vi "Get Plot to Fit.vi"(8 "error in (no error)":errorcluster, 9 "Plot Index":i32, 11 "XYGraph in":T2) -> (0 "error out":errorcluster, 1 "Plot Name":string, 2 "Y Array out":dbl[](array[numeric]), 3 "X Array out":dbl[](array[numeric]), 4 "Plot Color":u32, 5 "(Clipped) Plot Range":T1, 7 "Plot clipped?":bool)   [LabVIEW 2019]
uses:
  Graphs/XY Graph/XY Graph Refnum.ctl
  Graphs/Plot Range.ctl
  Histograms/Histogram Window.lvlib
  Graphs/XY Graph/XY Graph Add-Ons.lvlib
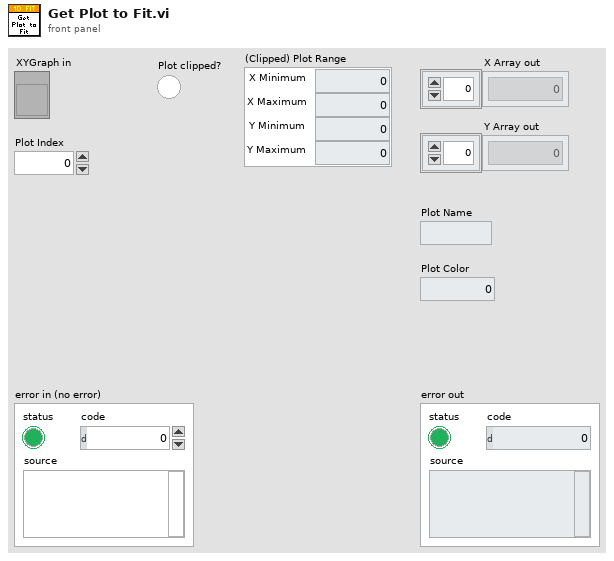
[diagram p1: front panel]
types:
  T1 = typedef "Plot Range.ctl" = cluster{"X Minimum":dbl, "X Maximum":dbl, "Y Minimum":dbl, "Y Maximum":dbl}
  T2 = typedef "XY Graph Add-Ons.lvlib/XY Graph Refnum.ctl" = refnum<vi>
  T3 = typedef "Histogram Bin Position.ctl" = enum16{"Left", "Center", "Right"}
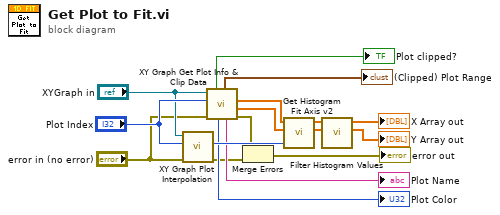
[diagram p0: block diagram]
diagram:
  n1 = call "XY Graph Plot Interpolation.vi"("error in (no error)"="error in (no error)", "Active Plot"="Plot Index", "XYGraph in"="XYGraph in") -> ("error out"=w3:errorcluster, "Bin Location"=w17:T3)  [unwired: 6 in, 1 out]
  n2 = call "XY Graph Get Plot Info & Clip Data.vi"("error in (no error)"="error in (no error)", "Plot index"="Plot Index", "XYGraph Ref in"="XYGraph in") -> ("error out"=w8:errorcluster, "Y Array"=w9:dbl[], "X Array"=w5:dbl[], "Plot Name"=→"Plot Name":string, "Plot Range"=→"(Clipped) Plot Range":T1, "Plot Color"=→"Plot Color":u32, "Plot Clipped?"=→"Plot clipped?":bool)  [unwired: 1 in, 1 out]
  n3 = Merge Errors(w8, w3) -> (→"error out":errorcluster)
  n4 = call "Get Histogram Fit Axis v2.vi"("Bin Location (Left)"=w17, "Histogram Values"=w9, "Histogram Axis"=w5) -> ("Ordered Axis Histogram Values"=w11:dbl[], "Ordered Histogram Axis"=w10:dbl[])  [unwired: 3 in, 4 out]
  n5 = call "Filter Histogram Values.vi"("Y Array in"=w11, "X Array in"=w10) -> ("Y Array out"=→"Y Array out":dbl[], "X Array out"=→"X Array out":dbl[])  [unwired: 7 in, 1 out]
